vi "showProgressBarClient(SubVI).vi"(8 "file size":i64, 11 "received":i64) -> (3 "progress":dbl(slide) scale=0.0..100.0)   [LabVIEW 2021]
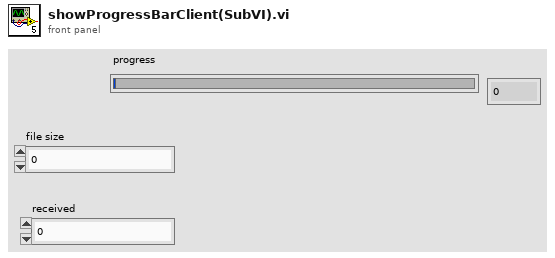
[diagram p1: front panel]
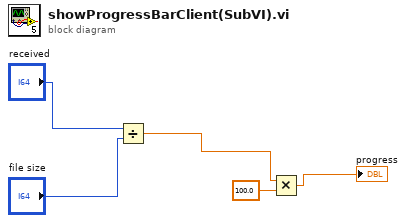
[diagram p0: block diagram]
diagram:
  n1 = Divide(x="received", y="file size") -> (x/y=w3:dbl)
  n2 = Multiply(x=w3, y=100.0) -> (x*y=→"progress":dbl)
